vi "RunPythonSideband.vi"(7 "Compiler Settings":T1={"Python Path"=path "C:/Users/LABadmin/.conda/envs/Jarvis/python.exe", "Main File"="mainscript.py", "Meta File"="metascript.txt", "Aux File"="auxscript.py", "Pre File"="metascript.txt"}, 8 "error in (no error)":errorcluster, 11 "params in":T2) -> (0 "error out":errorcluster, 3 "times array out":dbl[](array[numeric]))   [LabVIEW 2019]
uses:
  PulseCompiler/CompilerSettings.ctl
panel:
  out "standard output":string
  out "standard error":string
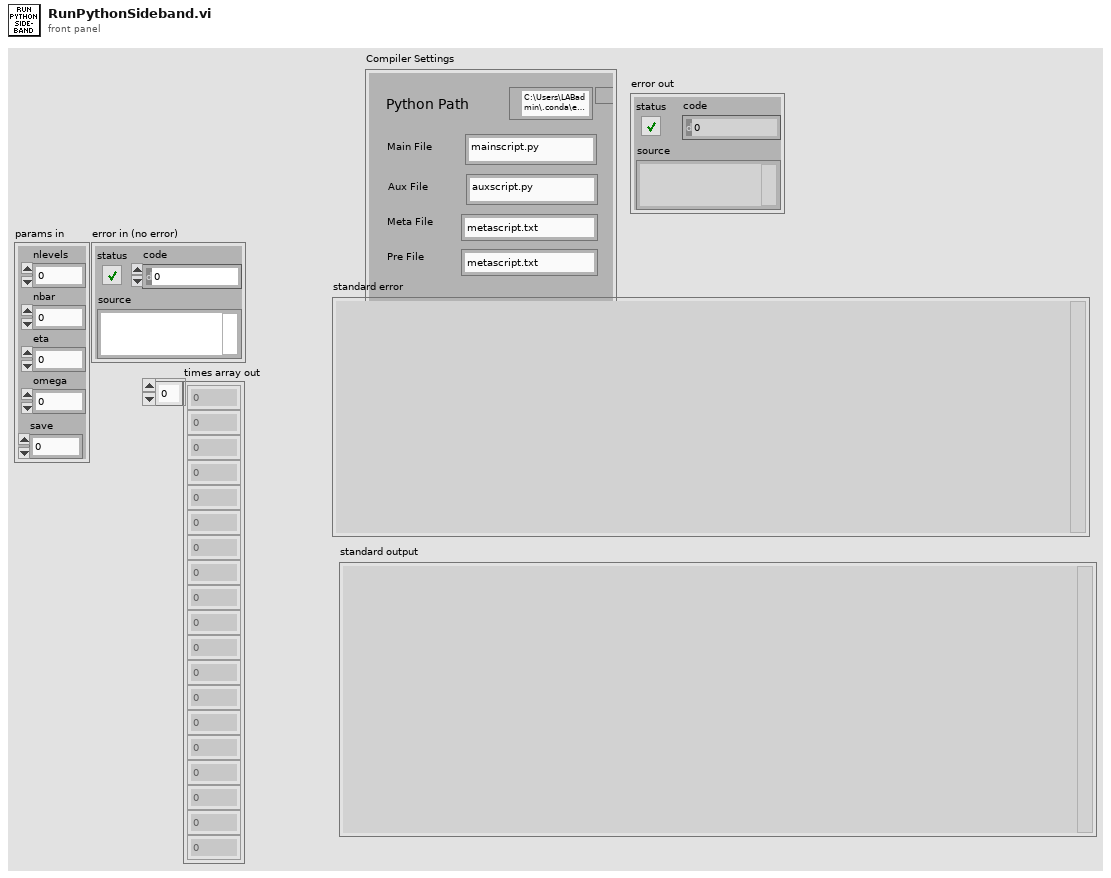
[diagram p1: front panel]
types:
  T1 = typedef "CompilerSettings.ctl" = cluster{"Python Path":path, "Main File":string, "Meta File":string, "Aux File":string, "Pre File":string}
  T2 = cluster{"nlevels":i32, "nbar":dbl, "eta":dbl, "omega":dbl, "save":dbl}
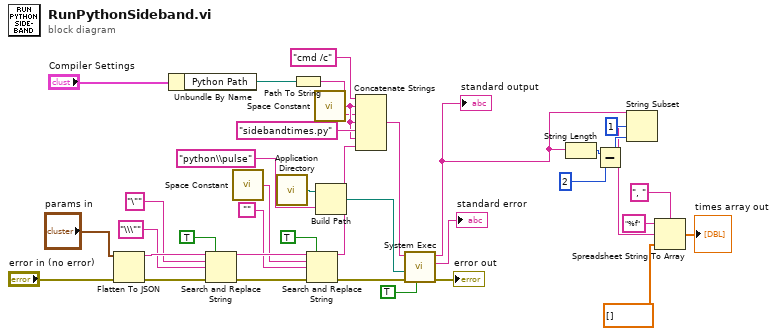
[diagram p0: block diagram]
diagram:
  n1 = Flatten To JSON(anything="params in", error in (no error)="error in (no error)") -> (JSON string=w33:string, 11:w30:errorcluster)  [unwired: 1 in]
  n2 = Unbundle By Name("Compiler Settings") -> ("Python Path"=w15:path)
  n3 = Search and Replace String(replace all?=TRUE ("replace all? (F)"), input string=w33, search string="\"", replace string="\\\"" ("replace string (\"\")"), error in=w30) -> (result string=w28:string, error out=w27:errorcluster)  [unwired: 3 in, 2 out]
  n4 = call <vilib>:"Space Constant.vi"() -> ("String"=w25:string)
  n5 = call <vilib>:"Application Directory.vi"() -> ("Application Directory"=w19:path)
  n6 = Path To String(path=w15) -> (string=w14:string)
  n7 = Search and Replace String(replace all?=TRUE ("replace all? (F)"), input string=w28, search string=w25, replace string="", error in=w27) -> (result string=w22:string, error out=w21:errorcluster)  [unwired: 3 in, 2 out]
  n8 = call <vilib>:"Space Constant.vi"() -> ("String"=w23:string)
  n9 = Build Path(base path=w19, name or relative path="python\\pulse") -> (appended path=w17:path)
  n10 = Concatenate Strings("cmd /c" ("string"), w23, w14, w23, "sidebandtimes.py", w23, w22) -> (w20:string)
  n11 = call <vilib>:"System Exec.vi"("run minimized? (F)"=TRUE, "error in (no error)"=w21, "working directory"=w17, "command line"=w20) -> ("error out"=→"error out":errorcluster, "standard error"=→"standard error":string, "standard output"=w6:string)  [unwired: 4 in, 1 out]
  "standard output" <- w6
  n12 = String Length(string=w6) -> (length=w5:i32)
  n13 = Subtract(x=w5, y=2) -> (x-y=w4:i32)
  n14 = String Subset(string=w6, offset (0)=1, length (rest)=w4) -> (substring=w2:string)
  n15 = Spreadsheet String To Array(delimiter (Tab)=", ", format string="%f", spreadsheet string=w2, array type (2D Dbl)=dbl[] []) -> (array=→"times array out":dbl[])
